vi "Controller Error.vi"(8 "error in (no error)":errorcluster, 11 "Data":variant) -> (0 "error out":errorcluster)   [LabVIEW 2018, in "Error Handler.lvlib"]
doc: "This subVI enqueues the named action in to the communications queue along with the input data."
uses:
  Error Handler.lvlib
  Private Controls/Module Data.ctl
  Private Controls/Module Action.ctl
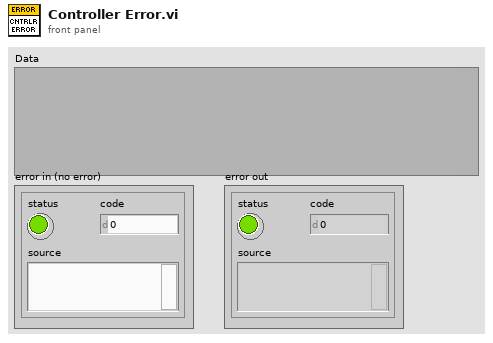
[diagram p1: front panel]
types:
  T1 = typedef "Error Handler.lvlib/Module Data.ctl" = cluster{"Data":variant, "Action":T2}
  T2 = typedef "Error Handler.lvlib/Module Action.ctl" = enum8{"Init", "Exit", "Controller Error", "UI1 Error", "UI2 Error", "UI3 Error", "File IO Error", "cRIO Error", "Calibration Error"}
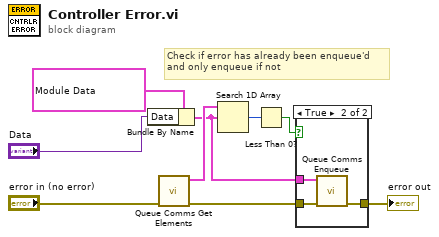
[diagram p0: block diagram]
diagram:
  # "Check if error has already been enqueue'd\nand only enqueue if not"
  n1 = Bundle By Name(cluster=T1 {"Data"=variant, "Action"=enum."Controller Error"} ("element"), "Data"="Data") -> (w3:T1)
  n2 = call "Queue Comms Get Elements.vi"("error in (no error)"="error in (no error)") -> ("error out"=w2:errorcluster, "elements"=w4:T1[])  [unwired: 9 in]
  n3 = Search 1D Array(1D array=w4, element=w3) -> (index of element=w5:i32)  [unwired: 1 in]
  n4 = Less Than 0?(x=w5) -> (x < 0?=w1:bool)
  n5 = case shown="True" w1 {
    tunnel: [w10 w13] -> w8
    tunnel: w3 -> [_ w12]
    tunnel: w2 -> [w10 w11]
    frame False {
    }
    frame True {
      n6 = call "Queue Comms Enqueue.vi"("error in (no error)"=w11, "element"=w12) -> ("error out"=w13:errorcluster)  [unwired: 9 in]
    }
  }
  "error out" <- w8
